vi "trivial_req.vi"() -> ()   [LabVIEW 2019]
uses:
  vi.lib/addons/zeromq/socket_type.ctl
  vi.lib/addons/zeromq/zmq_context.lvclass
  vi.lib/addons/zeromq/zmq_socket.lvclass
  vi.lib/addons/zeromq/zeromq.lvlib
panel:
  out "reply":string
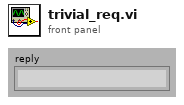
[diagram p1: front panel]
types:
  T1 = typedef "zeromq.lvlib/socket_type.ctl" = enum8{"ZMQ_PAIR", "ZMQ_PUB", "ZMQ_SUB", "ZMQ_REQ", "ZMQ_REP", "ZMQ_DEALER", "ZMQ_ROUTER", "ZMQ_PULL", "ZMQ_PUSH", "ZMQ_XPUB", "ZMQ_XSUB"}
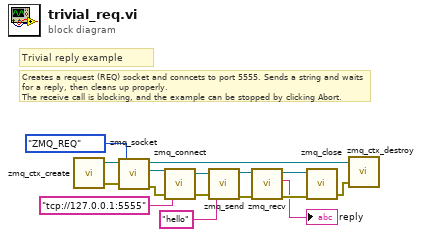
[diagram p0: block diagram]
diagram:
  # "Creates a request (REQ) socket and conncets to port 5555. Sends a string and waits for a reply, then cleans up properly.\nThe receive call is blocking, and the example can be stopped by clicking Abort."
  # "Trivial reply example"
  n1 = call "zmq_ctx_create.vi"() -> ("error out"=w6:errorcluster, "context out"=w16:refnum<class "zmq_context.lvclass">)  [unwired: 4 in]
  n2 = call "zmq_socket.vi"("error in"=w6, "socket type"=socket_type."ZMQ_REQ", "context in"=w16) -> ("error out"=w15:errorcluster, "socket out"=w14:refnum<class "zmq_socket.lvclass">, "context out"=w7:refnum<class "zmq_context.lvclass">)  [unwired: 2 in]
  n3 = call "zmq_connect.vi"("error in"=w15, "endpoint"="tcp://127.0.0.1:5555", "socket in"=w14) -> ("error out"=w13:errorcluster, "socket out"=w12:refnum<class "zmq_socket.lvclass">)  [unwired: 1 in]
  n4 = call "zmq_send.vi"("error in"=w13, "data"="hello", "socket in"=w12) -> ("error out"=w5:errorcluster, "socket out"=w11:refnum<class "zmq_socket.lvclass">)  [unwired: 4 in]
  n5 = call "zmq_recv.vi"("error in"=w5, "socket in"=w11) -> ("error out"=w10:errorcluster, "data"=→"reply":string, "socket out"=w9:refnum<class "zmq_socket.lvclass">)  [unwired: 3 in, 2 out]
  n6 = call "zmq_close.vi"("error in"=w10, "socket"=w9) -> ("error out"=w8:errorcluster)  [unwired: 3 in]
  n7 = call "zmq_ctx_destroy.vi"("error in"=w8, "context in"=w7) -> ()  [unwired: 3 in, 1 out]
